vi "PIDController_Pack_ErrorTolerance.vi"(9 "VelocityTolerance":dbl=9.9e+30, 11 "PositionTolerance":dbl=0.001) -> (3 "PID Error Tolerance":T1)   [LabVIEW 2019, in "Trajectory_Library.lvlib"]
doc: "Convience function to pack the input tolerance values into a data cluster that is used as input to the PID controller.\n\nInputs:\n - Position Tolerance -- Position tolerance in the same units as the PV and SP. (Default 0.001 )\n - Velocity Tolerance -- Velocity tolerance in the same units as the PV and SP.( Default 9.9E30 )"
uses:
  Trajectory_Library.lvlib
  PID_ERROR_TOLERANCE.ctl
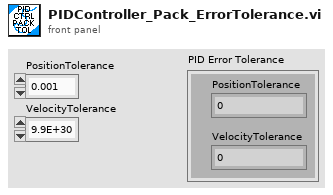
[diagram p1: front panel]
types:
  T1 = typedef "Trajectory_Library.lvlib/PID_ERROR_TOLERANCE.ctl" = cluster{"PositionTolerance":dbl, "VelocityTolerance":dbl}
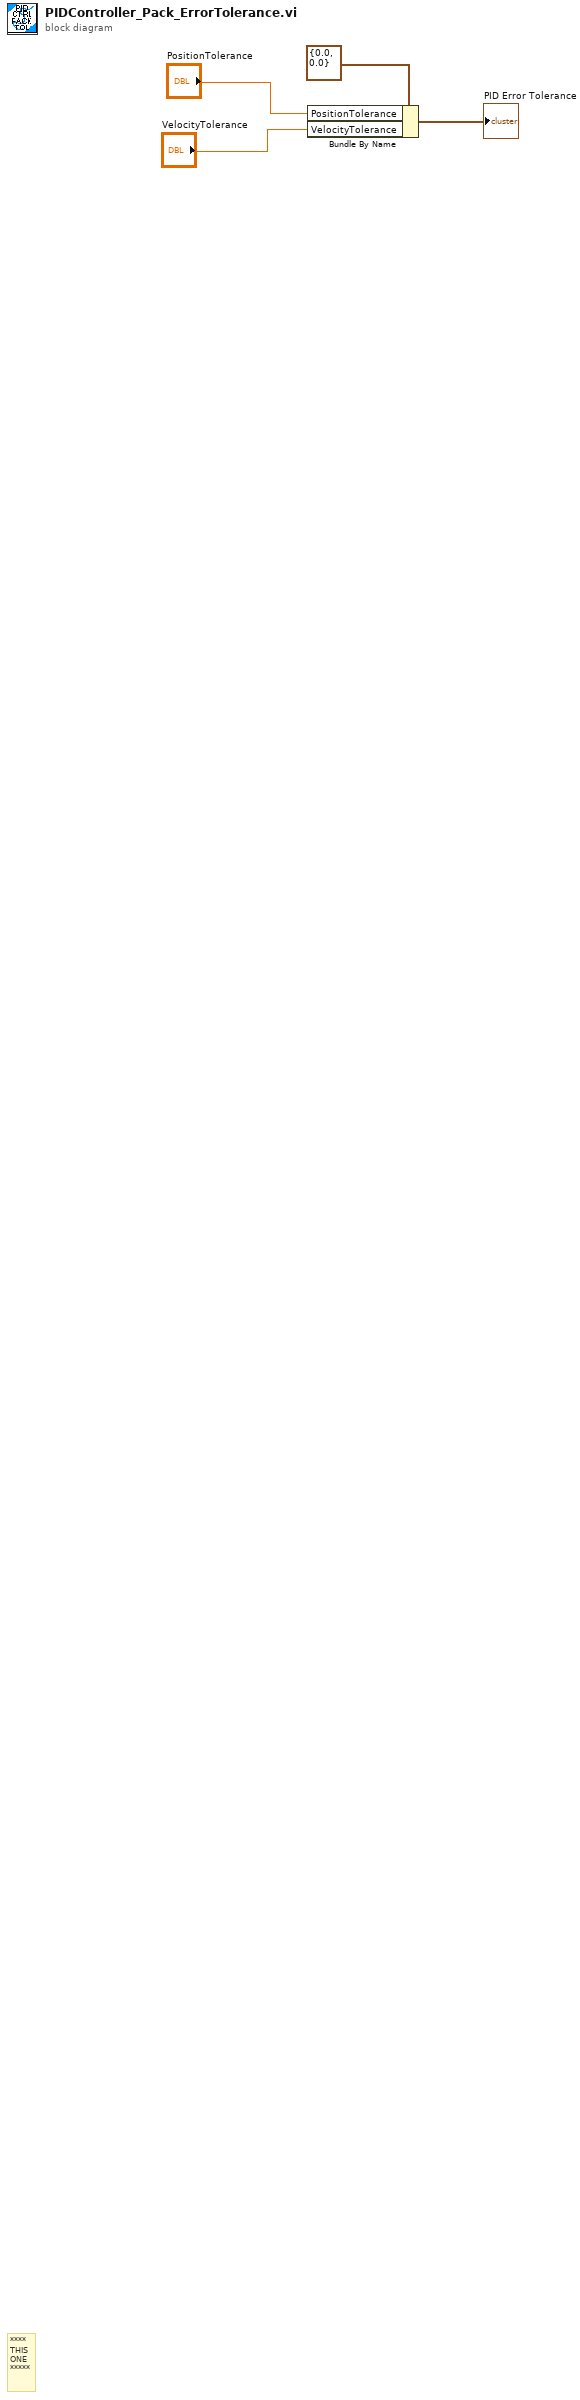
[diagram p0: block diagram]
diagram:
  # "****\nTHIS\nONE\n*****"
  n1 = Bundle By Name(cluster=T1 {"PositionTolerance"=0.0, "VelocityTolerance"=0.0} ("PID Error Tolerance"), "PositionTolerance"="PositionTolerance", "VelocityTolerance"="VelocityTolerance") -> (→"PID Error Tolerance":T1)
